vi "Call.vi"(6 "error in":errorcluster, 9 "FlatSequenceFrame in":refnum<class "FlatSequenceFrame.lvclass">) -> (0 "error out":errorcluster, 3 "FlatSequenceFrame out":refnum<class "FlatSequenceFrame.lvclass">, 4 "call":string)   [LabVIEW 2014, in "Raspberry Pi Compatible Compiler for LabVIEW.lvlib" / "FlatSequenceFrame.lvclass"]
uses:
  FlatSequenceFrame.lvclass
  Python/Parsing/ListTypesTD.ctl
  FlatSequenceFrame.lvclass/FlatSequenceFrame.ctl
  FlatSequenceInnerTunnel/FlatSequenceInnerTunnel.lvclass/FlatSequenceInnerTunnel.ctl
  FlatSequenceOuterTunnel/FlatSequenceOuterTunnel.lvclass/FlatSequenceOuterTunnel.ctl
  Terminal/Terminal.lvclass
  Python/Parsing/Python Functions.lvlib
  FlatSequenceOuterTunnel/FlatSequenceOuterTunnel.lvclass
  FlatSequenceInnerTunnel/FlatSequenceInnerTunnel.lvclass
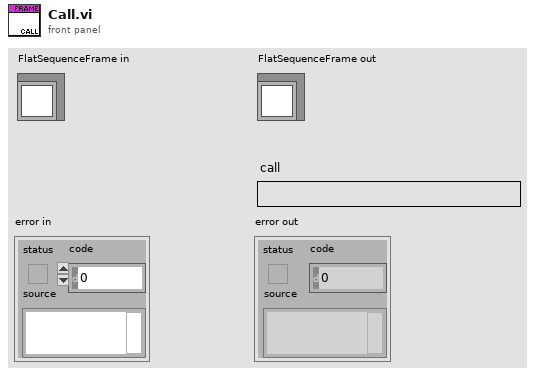
[diagram p1: front panel]
types:
  T1 = typedef "Raspberry Pi Compatible Compiler for LabVIEW.lvlib/Python Functions.lvlib/ListTypesTD.ctl" = enum16{"list", "tuple", "parameter list", "output list", "return values"}
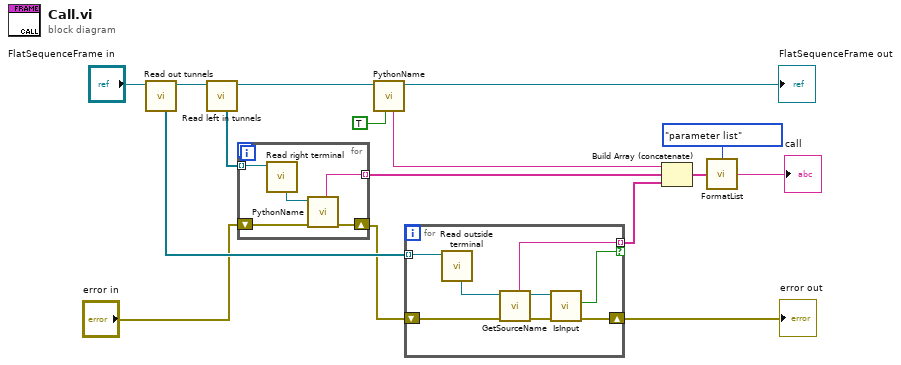
[diagram p0: block diagram]
diagram:
  n1 = call "Read out tunnels.vi"("FlatSequenceFrame in"="FlatSequenceFrame in") -> ("FlatSequenceFrame out"=w9:refnum<class "FlatSequenceFrame.lvclass">, "out tunnels"=w11:refnum<class "FlatSequenceOuterTunnel.lvclass">[])  [unwired: 7 in]
  n2 = call "Read left in tunnels.vi"("FlatSequenceFrame in"=w9) -> ("FlatSequenceFrame out"=w10:refnum<class "FlatSequenceFrame.lvclass">, "left in tunnels"=w12:refnum<class "FlatSequenceInnerTunnel.lvclass">[])  [unwired: 7 in]
  n3 = for {
    tunnel: w12 -> [w21] mode=indexing
    shift-right: [w17] -> w7
    shift-left: "error in" -> [w20]
    tunnel: [w18] -> w6 mode=indexing
    n4 = call "Read right terminal.vi"("FlatSequenceInnerTunnel in"=w21) -> ("right terminal"=w19:refnum<class "Terminal.lvclass">)  [unwired: 7 in, 1 out]
    n5 = call-dynamic "PythonName.vi"("error in"=w20, "Terminal in"=w19) -> ("error out"=w17:errorcluster, "name"=w18:string)  [unwired: 6 in, 2 out]
  }
  n6 = call-dynamic "PythonName.vi"("add self"=TRUE, "FlatSequenceFrame in"=w10) -> ("FlatSequenceFrame out"=→"FlatSequenceFrame out":refnum<class "FlatSequenceFrame.lvclass">, "name"=w13:string)  [unwired: 6 in, 2 out]
  n7 = for {
    tunnel: w11 -> [w29] mode=indexing
    shift-right: [w24] -> w3
    shift-left: w7 -> [w27]
    tunnel: [w25] -> w5 mode=indexing if=w23
    n8 = call "Read outside terminal.vi"("FlatSequenceInnerTunnel in"=w29) -> ("outside terminal"=w28:refnum<class "Terminal.lvclass">)  [unwired: 7 in, 1 out]
    n9 = call "GetSourceName.vi"("error in"=w27, "Terminal in"=w28) -> ("error out"=w26:errorcluster, "Terminal out"=w22:refnum<class "Terminal.lvclass">, "source"=w25:string)  [unwired: 5 in]
    n10 = call-dynamic "IsInput.vi"("error in"=w26, "Terminal in"=w22) -> ("error out"=w24:errorcluster, "input"=w23:bool)  [unwired: 5 in, 1 out]
  }
  "error out" <- w3
  n11 = Build Array (concatenate)(w13, w6, w5) -> (w14:string[])
  n12 = call "FormatList.vi"("values"=w14, "type"=ListTypesTD."parameter list") -> ("python object"=→"call":string)
